vi "CRYPEAQ NCorr.vi"(8 "M":dbl, 9 "NL":dbl, 10 "D":dbl[](array[numeric]), 11 "C":dbl[](array[numeric])) -> (3 "Cn":dbl[](array[numeric]))   [LabVIEW 2013]
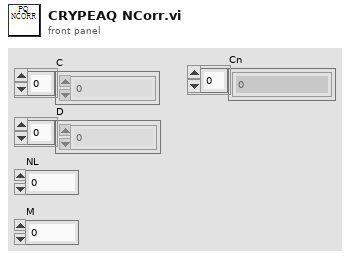
[diagram p1: front panel]
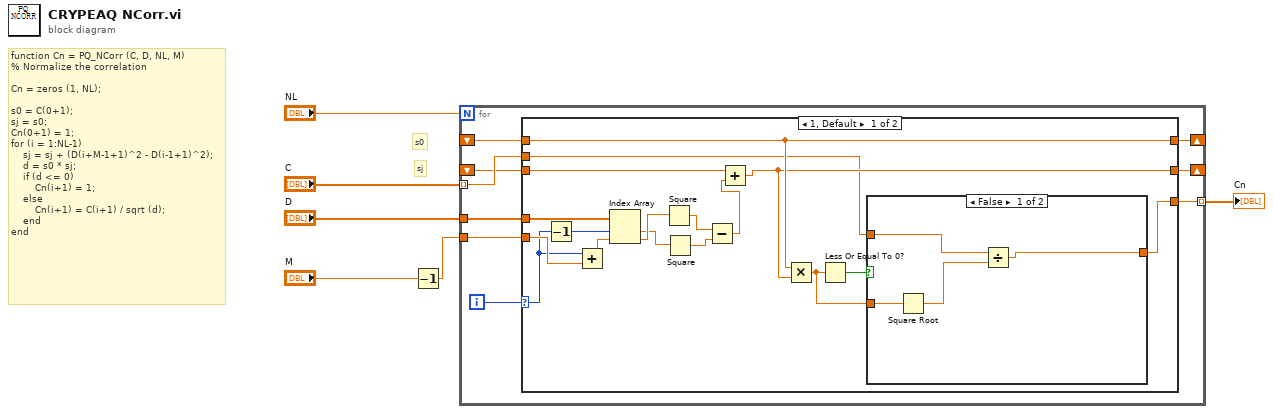
[diagram p0: block diagram]
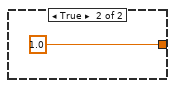
[diagram p2: hidden frame]
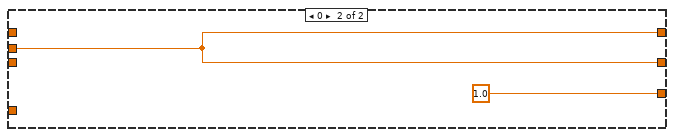
[diagram p3: hidden frame]
diagram:
  # "sj"
  # "s0"
  # "function Cn = PQ_NCorr (C, D, NL, M)\n% Normalize the correlation\n\nCn = zeros (1, NL);\n\ns0 = C(0+1);\nsj = s0;\nCn(0+1) = 1;\nfor (i = 1:NL-1)\n    sj = sj + (D(i+M-1+1)^2 - D(i-1+1)^2);\n    d = s0 * sj;\n    if (d <= 0)\n        Cn(i+1) = 1;\n    else\n        Cn(i+1) = C(i+1) / sqrt (d);\n    end\nend"
  n1 = Decrement(x="M") -> (x-1=w6:dbl)
  n2 = for {
    N: "NL" -> [_]
    tunnel: [w14] -> w1 mode=indexing
    tunnel: "C" -> [w13] mode=indexing
    tunnel: "D" -> [w12]
    shift-right: [w11] -> _
    shift-left: _ -> [w7]
    shift-right: [w10] -> _
    shift-left: _ -> [w9]
    tunnel: w6 -> [w8]
    i -> [w15]
    n3 = case shown="1, Default" w15 {
      selector: w15 -> [w28 _]
      tunnel: [w18 1.0] -> w14
      tunnel: w13 -> [w17 w38]
      tunnel: w12 -> [w31 _]
      tunnel: [w21 w38] -> w11
      tunnel: [w20 w38] -> w10
      tunnel: w9 -> [w32 _]
      tunnel: w8 -> [w29 _]
      tunnel: w7 -> [w21 _]
      frame 1, Default {
        n4 = Decrement(x=w28) -> (x-1=w30:i32)
        n5 = Add(x=w28, y=w29) -> (x+y=w27:dbl)
        n6 = Index Array(array=w31, index #1=w30, index #2=w27) -> (element #1=w25:dbl, element #2=w26:dbl)
        n7 = Square(x=w26) -> (x^2=w24:dbl)
        n8 = Square(x=w25) -> (x^2=w23:dbl)
        n9 = Subtract(x=w24, y=w23) -> (x-y=w22:dbl)
        n10 = Add(x=w32, y=w22) -> (x+y=w20:dbl)
        n11 = Multiply(x=w21, y=w20) -> (x*y=w16:dbl)
        n12 = Less Or Equal To 0?(x=w16) -> (x <= 0?=w19:bool)
        n13 = case shown="False" w19 {
          tunnel: [w33 1.0] -> w18
          tunnel: w17 -> [w36 _]
          tunnel: w16 -> [w35 _]
          frame False {
            n14 = Square Root(x=w35) -> (sqrt(x)=w34:dbl)
            n15 = Divide(x=w36, y=w34) -> (x/y=w33:dbl)
          }
          frame True {
          }
        }
      }
      frame 0 {
      }
    }
  }
  "Cn" <- w1
